vi "周期设置_氨氮.vi"() -> ()   [LabVIEW 2016, in "斯坦道氨氮.lvlib"]
uses:
  <vilib>/Utility/miscctls.llb/LVPointTypeDef.ctl
  <vilib>/Utility/config.llb/NI_LVConfig.lvlib
panel:
  in  "运行周期":T1={"运行模式"=enum."维护模式", "质控频次"=enum."关闭", "空白核查时间"=2, "跨度核查时间"=6, "24H周期设置"=[]} {"跨度核查时间" items=["00H", "01H", "02H", "03H", "04H", "05H", "06H", "07H", "08H", "09H", "10H", "11H", "12H", "13H", "14H", "15H", "16H", "17H", "18H", "19H", "20H", "21H", "22H", "23H", "关闭"]; "空白核查时间" items=["00H", "01H", "02H", "03H", "04H", "05H", "06H", "07H", "08H", "09H", "10H", "11H", "12H", "13H", "14H", "15H", "16H", "17H", "18H", "19H", "20H", "21H", "22H", "23H", "关闭"]}
  # "运行模式："
  # "质控频次："
  # "空白核查时间："
  # "跨度核查时间："
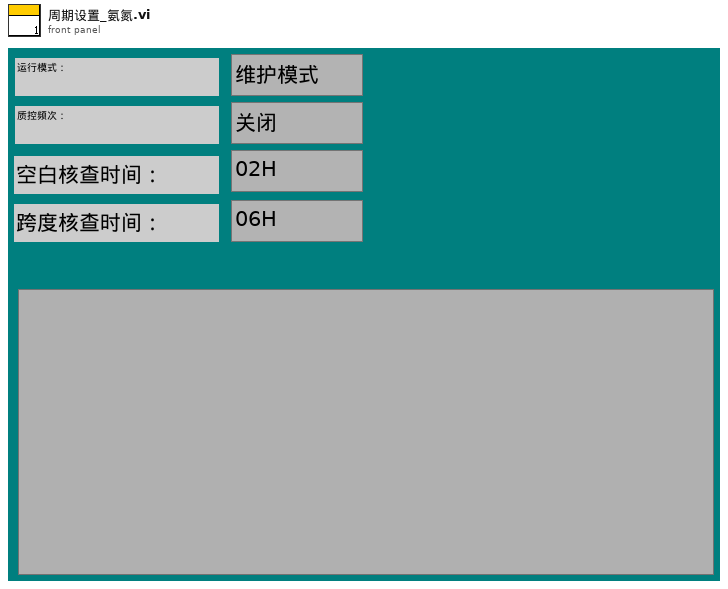
[diagram p1: front panel]
types:
  T1 = cluster{"运行模式":enum16{"维护模式", "常规模式", "应急模式", "质控模式"}, "质控频次":enum16{"关闭", "每天", "星期一", "星期二", "星期三", "星期四", "星期五", "星期六", "星期日"}, "空白核查时间":u16, "跨度核查时间":u16, "24H周期设置":bool[]}
  T2 = typedef "LVPointTypeDef.ctl" = cluster{"Horizontal":i16, "Vertical":i16}
  T3 = enum16{"启动测量", "标样核查", "零点核查", "跨度核查", "空白测试", "平行样测试", "加标回收", "空白校准", "标样校准", "初始化（清洗）", "停止测试", "仪器重启", "校时", "模式设置", "测量间隔设置"}
  T4 = enum16{"关闭", "每天", "星期一", "星期二", "星期三", "星期四", "星期五", "星期六", "星期日"}
  T5 = typedef "LVDateTimeRec.ctl" = cluster{"秒数的小数部分":dbl, "秒":i32, "分":i32, "时":i32, "日":i32, "月":i32, "年":i32, "天数（周）":i32, "天数（年）":i32, "DST":i32}
  T6 = enum32{"Bad", "Idle", "Run top level", "Running"}
  T7 = cluster{"水样测试量程模式":enum16{"H", "L", "AUTO"}, "空白核查量程模式":enum16{"H", "L", "AUTO"}, "跨度核查量程模式":enum16{"H", "L", "AUTO"}}
  T8 = typedef "NI_LVConfig.lvlib/Config Data RefNum.ctl" = refnum<k1>
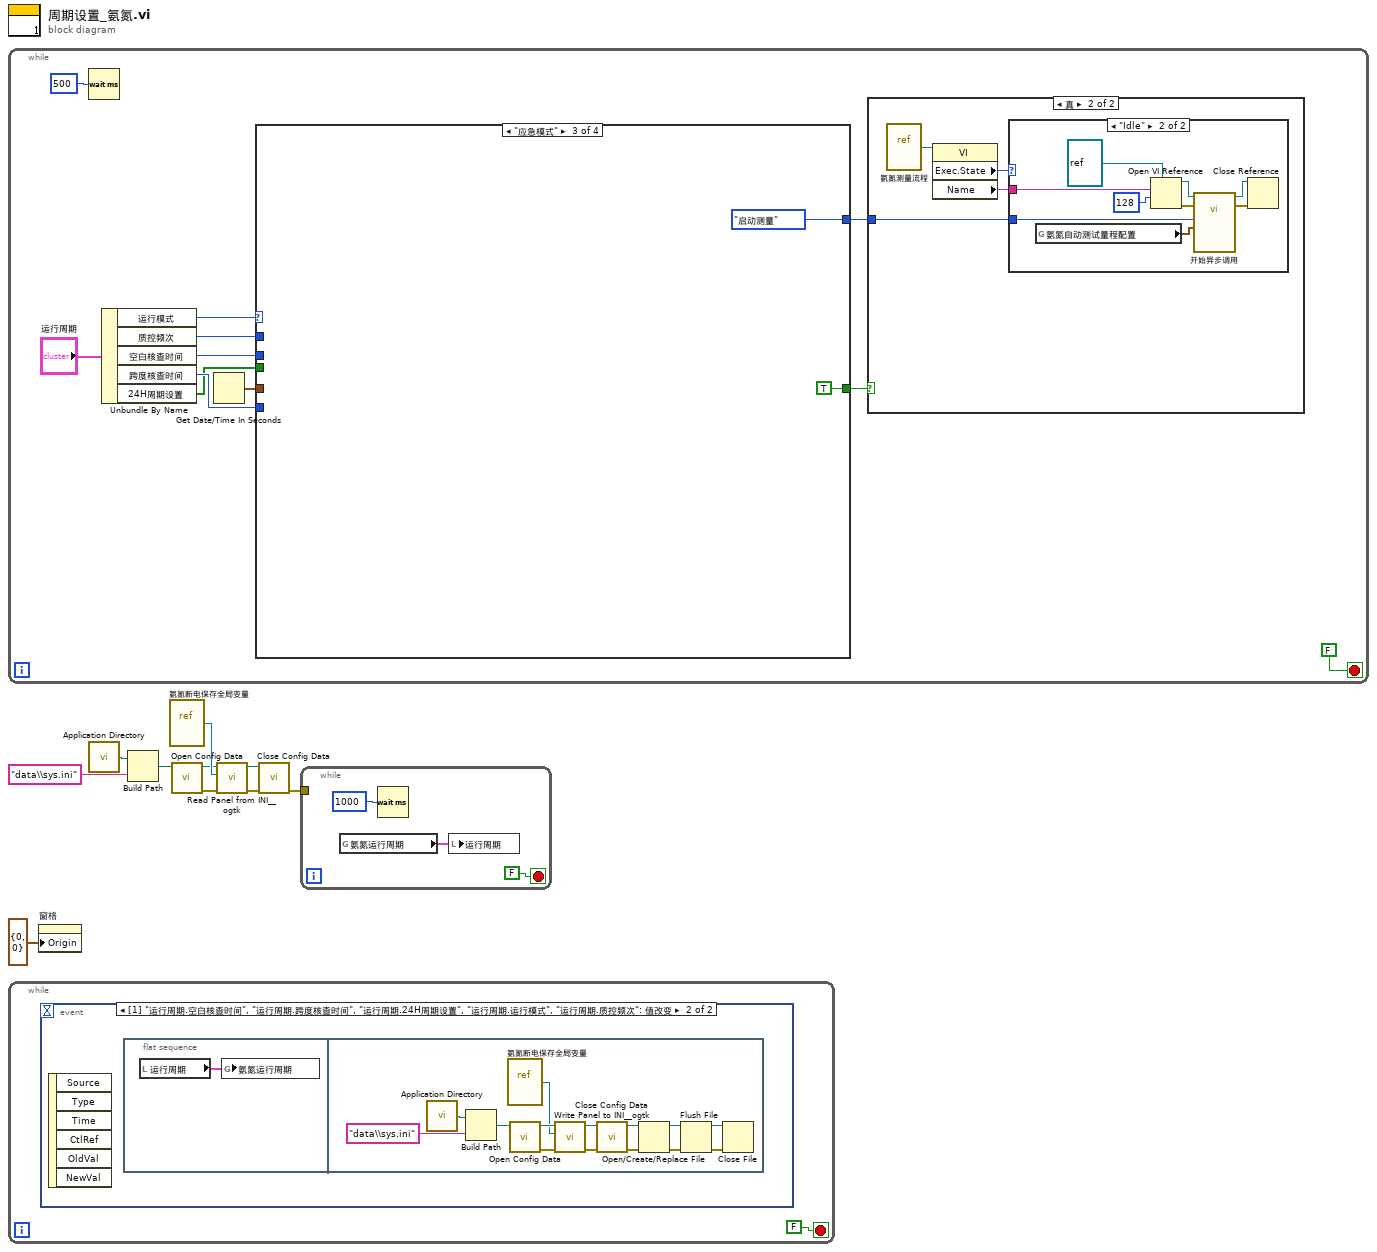
[diagram p0: block diagram]
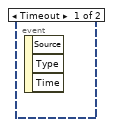
[diagram p2: hidden frame]
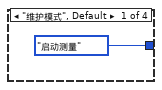
[diagram p5: hidden frame]
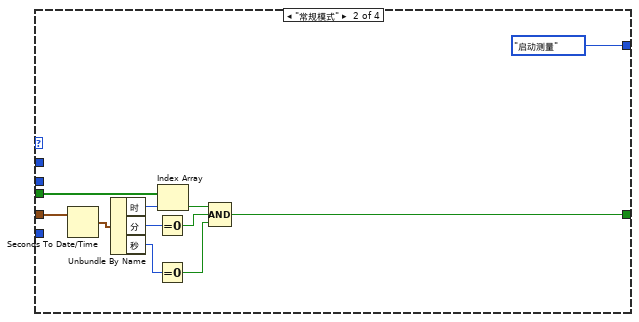
[diagram p6: hidden frame]
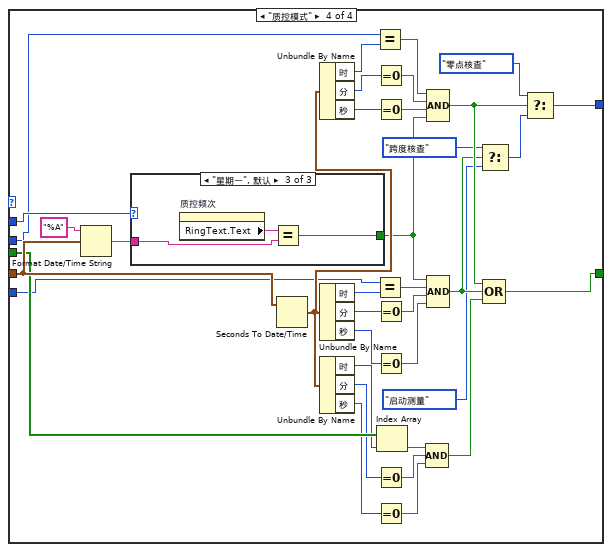
[diagram p7: hidden frame]
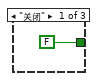
[diagram p8: hidden frame]
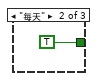
[diagram p9: hidden frame]
diagram:
  n1 = while {
    stop <- FALSE stop-if-true
    n2 = Wait (ms)(milliseconds to wait=u32 500 ("等待时间（毫秒）")) -> ()  [unwired: 1 out]
    n3 = Unbundle By Name("运行周期") -> ("运行模式"=w15:enum16{"维护模式", "常规模式", "应急模式", "质控模式"}, "质控频次"=w14:T4, "空白核查时间"=w13:u16, "跨度核查时间"=w12:u16, "24H周期设置"=w11:bool[])
    n4 = Get Date/Time In Seconds() -> (seconds since 1Jan1904=w21:timestamp)
    n5 = case shown="\"应急模式\"" w15 {
      tunnel: w21 -> [_ w46 _ w84]
      tunnel: w11 -> [_ w43 _ w81]
      tunnel: [_ w37 TRUE w61] -> w18
      tunnel: [T3."启动测量" ("控制命令") T3."启动测量" ("控制命令") T3."启动测量" ("控制命令") w57] -> w17
      tunnel: w14 -> [_ _ _ w54]
      tunnel: w13 -> [_ _ _ w53]
      tunnel: w12 -> [_ _ _ w52]
      frame "维护模式", Default {
      }
      frame "常规模式" {
        n6 = Seconds To Date/Time(time stamp (now)=w46) -> (date time rec=w45:T5)  [unwired: 1 in]
        n7 = Unbundle By Name(w45) -> ("时"=w44:i32, "分"=w42:i32, "秒"=w41:i32)
        n8 = Equal To 0?(x=w42) -> (x = 0?=w39:bool)
        n9 = Equal To 0?(x=w41) -> (x = 0?=w38:bool)
        n10 = Index Array(array=w43, index=w44) -> (element=w40:bool)
        n11 = Compound Arithmetic op=AND ("复合运算")(w40, w39, w38) -> (w37:bool)
      }
      frame "应急模式" {
      }
      frame "质控模式" {
        n12 = Format Date/Time String(time format string (%c)="%A" ("时间格式字符串(%c)"), seconds (now)=w84) -> (date/time string=w82:string)  [unwired: 1 in]
        n13 = case shown="\"星期一\", 默认" w54 {
          tunnel: w82 -> [_ _ w88]
          tunnel: [FALSE TRUE w87] -> w55
          frame "关闭" {
          }
          frame "每天" {
          }
          frame "星期一", Default {
            n14 = property on="质控频次" class="Enum (严格)"() -> ("RingText.Text"=w89:string)  [unwired: 2 in, 2 out]
            n15 = Equal?(x=w89, y=w88) -> (x = y?=w87:bool)
          }
        }
        n16 = Seconds To Date/Time(time stamp (now)=w84) -> (date time rec=w65:T5)  [unwired: 1 in]
        n17 = Unbundle By Name(w65) -> ("时"=w74:i32, "分"=w73:i32, "秒"=w72:i32)
        n18 = Unbundle By Name(w65) -> ("时"=w66:i32, "分"=w67:i32, "秒"=w68:i32)
        n19 = Unbundle By Name(w65) -> ("时"=w80:i32, "分"=w78:i32, "秒"=w76:i32)
        n20 = Equal?(x=w53, y=w74) -> (x = y?=w71:bool)
        n21 = Equal?(x=w52, y=w66) -> (x = y?=w64:bool)
        n22 = Equal To 0?(x=w73) -> (x = 0?=w70:bool)
        n23 = Equal To 0?(x=w72) -> (x = 0?=w69:bool)
        n24 = Equal To 0?(x=w67) -> (x = 0?=w63:bool)
        n25 = Equal To 0?(x=w68) -> (x = 0?=w62:bool)
        n26 = Equal To 0?(x=w78) -> (x = 0?=w77:bool)
        n27 = Equal To 0?(x=w76) -> (x = 0?=w75:bool)
        n28 = Index Array(array=w81, index=w80) -> (element=w79:bool)
        n29 = Compound Arithmetic op=AND ("复合运算")(w79, w77, w75) -> (w56:bool)
        n30 = Compound Arithmetic op=AND ("复合运算")(w71, w70, w69, w55) -> (w60:bool)
        n31 = Compound Arithmetic op=AND ("复合运算")(w55, w64, w63, w62) -> (w59:bool)
        n32 = Select(t=T3."跨度核查" ("控制命令"), s=w59, f=T3."启动测量" ("控制命令")) -> (s? t:f=w58:T3)
        n33 = Compound Arithmetic op=OR ("复合运算")(w60, w59, w56) -> (w61:bool)
        n34 = Select(t=T3."零点核查" ("控制命令"), s=w60, f=w58) -> (s? t:f=w57:T3)
      }
    }
    n35 = case shown="真" w18 {
      tunnel: w17 -> [_ w22]
      frame False {
      }
      frame True {
        n36 = vi-ref "氨氮测量流程.vi"() -> (w23:refnum<vi>)
        n37 = property class="VI"(reference=w23) -> ("Exec.State"=w25:T6, "Name"=w24:string)  [unwired: 1 in, 2 out]
        n38 = case shown="\"Idle\"" w25 {
          tunnel: w24 -> [_ w30]
          tunnel: w22 -> [_ w26]
          frame "Bad", Default {
          }
          frame "Idle" {
            n39 = global read "氨氮断电保存全局变量.vi" "氨氮自动测试量程配置"() -> (w28:T7)
            n40 = Open VI Reference(type specifier VI Refnum (for type only)=refnum<vi> refnum, vi path=w30, options=128 ("选项")) -> (vi reference=w31:refnum<vi>, error out=w32:errorcluster)  [unwired: 3 in]
            n41 = call-by-ref "开始异步调用"(reference=w31, error in=w32, "总磷量程模式"=w28, "控制命令"=w26) -> (reference out=w33:refnum<vi>, error out=w34:errorcluster)  [unwired: 10 in]
            n42 = Close Reference(reference=w33, error in (no error)=w34) -> ()  [unwired: 1 out]
          }
        }
      }
    }
  }
  n43 = while {
    stop <- FALSE stop-if-true
    n44 = event shown="[1] \"运行周期.空白核查时间\", \"运行周期.跨度核查时间\", \"运行周期.24H周期设置\", \"运行周期.运行模式\", \"运行周期.质控频次\": 值改变" {
      selector: _ -> [_ _]
      dyn-events: _ -> [_ _]
      timeout: _ -> [_ _]
      event Timeout {
        n45 = event-data() -> ()  [unwired: 1 in, 3 out]
      }
      event "运行周期.空白核查时间", "运行周期.跨度核查时间", "运行周期.24H周期设置", "运行周期.运行模式", "运行周期.质控频次": Value Change {
        n46 = event-data() -> ()  [unwired: 1 in, 6 out]
        n47 = flat-sequence {
          frame #0 {
            n48 = local read "运行周期"() -> (w91:T1)
            n49 = global write "氨氮断电保存全局变量.vi" "氨氮运行周期"(w91) -> ()
          }
          frame #1 {
            n50 = call <vilib>:"Application Directory.vi"() -> ("Application Directory"=w105:path)
            n51 = Build Path(base path=w105, name or relative path="data\\sys.ini" ("名称或相对路径")) -> (appended path=w103:path)
            n52 = vi-ref "氨氮断电保存全局变量.vi"() -> (w101:refnum<vi>)
            n53 = call <vilib>:"Open Config Data.vi"("configuration file path"=w103) -> ("error out"=w99:errorcluster, "refnum"=w102:T8)  [unwired: 8 in, 1 out]
            n54 = call <userlib>:"Write Panel to INI__ogtk.vi"("error in (no error)"=w99, "VI ref"=w101, "refnum"=w102) -> ("error out"=w98:errorcluster, "refnum out"=w100:T8)  [unwired: 7 in]
            n55 = call <vilib>:"Close Config Data.vi"("error in (no error)"=w98, "refnum"=w100) -> ("error out"=w93:errorcluster, "file path"=w92:path)  [unwired: 8 in]
            n56 = Open/Create/Replace File(file path (use dialog)=w92, error in=w93) -> (refnum out=w96:refnum<file>, error out=w97:errorcluster)  [unwired: 4 in, 1 out]
            n57 = Flush File(refnum=w96, error in=w97) -> (refnum out=w95:refnum<file>, error out=w94:errorcluster)
            n58 = Close File(refnum=w95, error in=w94) -> ()  [unwired: 2 out]
          }
        }
      }
    }
  }
  n59 = property on="窗格" class="Pane"("Origin"=T2 {"Horizontal"=0, "Vertical"=0} ("原点")) -> ()  [unwired: 2 in, 2 out]
  n60 = call <vilib>:"Application Directory.vi"() -> ("Application Directory"=w3:path)
  n61 = Build Path(base path=w3, name or relative path="data\\sys.ini" ("名称或相对路径")) -> (appended path=w5:path)
  n62 = vi-ref "氨氮断电保存全局变量.vi"() -> (w7:refnum<vi>)
  n63 = call <vilib>:"Open Config Data.vi"("configuration file path"=w5) -> ("error out"=w9:errorcluster, "refnum"=w6:T8)  [unwired: 8 in, 1 out]
  n64 = call <userlib>:"Read Panel from INI__ogtk.vi"("error in (no error)"=w9, "VI ref"=w7, "refnum"=w6) -> ("error out"=w10:errorcluster, "refnum out"=w8:T8)  [unwired: 7 in]
  n65 = call <vilib>:"Close Config Data.vi"("error in (no error)"=w10, "refnum"=w8) -> ("error out"=w2:errorcluster)  [unwired: 8 in, 1 out]
  n66 = while {
    tunnel: w2 -> [_]
    stop <- FALSE stop-if-true
    n67 = global read "氨氮断电保存全局变量.vi" "氨氮运行周期"() -> (w106:T1)
    n68 = Wait (ms)(milliseconds to wait=u32 1000 ("等待时间（毫秒）")) -> ()  [unwired: 1 out]
    n69 = local write "运行周期"(w106) -> ()
  }
